vi "Parameters.vi"(8 "error in (no error)":errorcluster, 11 "Template Test Case In":refnum<class "02_FeatureDetectionAprilTag.lvclass">) -> (0 "error out":errorcluster, 2 "Parameters":T1(array[cluster]))   [LabVIEW 2020, in "test.lvlib" / "02_FeatureDetectionAprilTag.lvclass"]
doc: "This VI defines the parameters used for execution. When LUnit runs the test case, it will run it once for every parameter in the array and collect the results.\n\nDuring test execution, the parameters are available in the class wire within the test VI."
uses:
  02_FeatureDetectionAprilTag.lvclass
  C:/Program Files (x86)/National Instruments/LabVIEW 2020/vi.lib/Astemes/LUnit Parameterized/Parameterized Test Case/Parameterized Test Case.lvclass
  <vilib>/Astemes/LUnit Parameterized/Parameterized Test Case/Parameterized Test Case.lvclass
  common/Quad Corners.ctl
  common/Image Point (Float).ctl
  02_FeatureDetectionAprilTag.lvclass/02_FeatureDetectionAprilTag.ctl
  common/common.lvlib
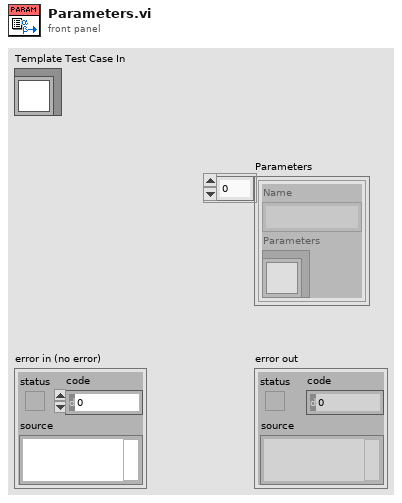
[diagram p1: front panel]
types:
  T1 = cluster{"Name":string, "Parameters":refnum<class "Parameterized Test Case.lvclass">}[]
  T2 = typedef "common.lvlib/Quad Corners.ctl" = cluster{"Bottom Left":T3, "Bottom Right":T3, "Top Right":T3, "Top Left":T3}
  T3 = typedef "common.lvlib/Image Point (Float).ctl" = cluster{"x":dbl, "y":dbl}
  T4 = cluster{string, cluster{"Family":enum8{"tag16h5", "tag25h9", "tag36h11", "tagCircle21h7", "tagCircle49h12", "tagCustom48h12", "tagStandard41h12", "tagStandard52h13"}, "Corners":T2}}[]
  T5 = cluster{"Scenario":string, "Parameters":refnum<class "02_FeatureDetectionAprilTag.lvclass">}[]
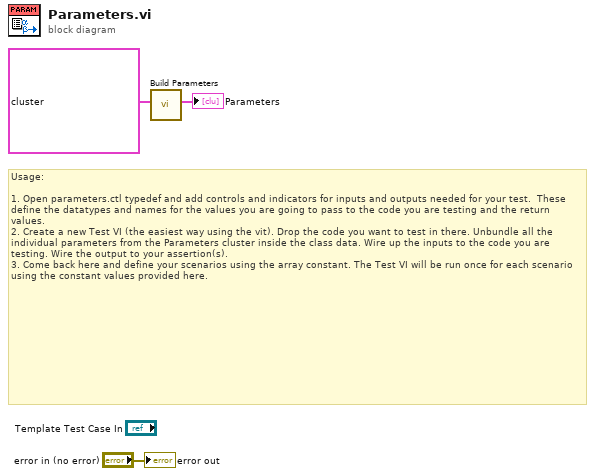
[diagram p0: block diagram]
diagram:
  # "Usage:\n\n1. Open parameters.ctl typedef and add controls and indicators for inputs and outputs needed for your test.  These define the datatypes and names for the values you are going to pass to the code you are testing and the return values.\n2. Create a new Test VI (the easiest way using the vit). Drop the code you want to test in there. Unbundle all the individual parameters from the Parameters cluster inside the class data. Wire up the inputs to the code you are testing. Wire the output to your assertion(s).\n3. Come back here and define your scenarios using the array constant. The Test VI will be run once for each scenario using the constant values provided here."
  n1 = call "Build Parameters.vi"("Scenarios In"=T4 [{"tag16h5", {"Family"=enum."tag16h5", "Corners"={"Bottom Left"={"x"=4.000000000000001, "y"=28.000000000000004}, "Bottom Right"={"x"=28.000000000000007, "y"=28.0}, "Top Right"={"x"=28.0, "y"=3.999999523162839}, "Top Left"={"x"=3.9999999999999973, "y"=4.000000476837156}}}}, {"tag25h9", {"Family"=enum."tag25h9", "Corners"={"Bottom Left"={"x"=4.000000000000001, "y"=32.00000000000001}, "Bottom Right"={"x"=32.00000000000001, "y"=31.999999999999996}, "Top Right"={"x"=31.999999999999996, "y"=3.9999992847442614}, "Top Left"={"x"=3.9999999999999973, "y"=4.0000004768371635}}}}, {"tag36h11", {"Family"=enum."tag36h11", "Corners"={"Bottom Left"={"x"=4.0, "y"=36.00000000000001}, "Bottom Right"={"x"=36.0, "y"=35.99999999999999}, "Top Right"={"x"=35.99999999999999, "y"=3.999999284744256}, "Top Left"={"x"=3.999999999999993, "y"=4.0000004768371635}}}}, {"tagCircle21h7", {"Family"=enum."tagCircle21h7", "Corners"={"Bottom Left"={"x"=12.000000000000002, "y"=32.0}, "Bottom Right"={"x"=32.0, "y"=32.0}, "Top Right"={"x"=32.0, "y"=11.999999999999998}, "Top Left"={"x"=11.999999999999998, "y"=12.000000000000002}}}}, {"tagCircle49h12", {"Family"=enum."tagCircle49h12", "Corners"={"Bottom Left"={"x"=16.0, "y"=36.0}, "Bottom Right"={"x"=36.0, "y"=36.0}, "Top Right"={"x"=36.0, "y"=15.999999999999998}, "Top Left"={"x"=15.999999999999998, "y"=16.0}}}}, {"tagCustom48h12", {"Family"=enum."tagCustom48h12", "Corners"={"Bottom Left"={"x"=12.000000000000002, "y"=36.0}, "Bottom Right"={"x"=36.0, "y"=36.0}, "Top Right"={"x"=36.0, "y"=12.000000953674311}, "Top Left"={"x"=11.999999999999998, "y"=11.999999046325682}}}}, {"tagStandard41h12", {"Family"=enum."tagStandard41h12", "Corners"={"Bottom Left"={"x"=12.000000000000002, "y"=32.0}, "Bottom Right"={"x"=32.0, "y"=32.0}, "Top Right"={"x"=32.0, "y"=11.999999999999998}, "Top Left"={"x"=11.999999999999998, "y"=12.000000000000002}}}}, {"tagStandard52h13", {"Family"=enum."tagStandard52h13", "Corners"={"Bottom Left"={"x"=12.000000000000002, "y"=36.0}, "Bottom Right"={"x"=36.0, "y"=36.0}, "Top Right"={"x"=36.0, "y"=12.000000953674311}, "Top Left"={"x"=11.999999999999998, "y"=11.999999046325682}}}}] ("appended array")) -> ("Scenarios out"=→"Parameters":T5)  [unwired: 10 in]
  "error out" <- "error in (no error)"
